vi "hse-application_SetApplicationVersion.vi"(8 "error in":errorcluster, 10 "Application Version History":string, 11 "Application Version Number":string) -> (0 "error out":errorcluster)   [LabVIEW 2020, in "hse-application.lvclass"]
doc: "Stores the version number of the application for later usage (display, logging, ...).\n\n\n\n____\nHAMPEL SOFTWARE ENGINEERING v3.8.0 (2023-12-18 14:41)"
uses:
  hse-application.lvclass
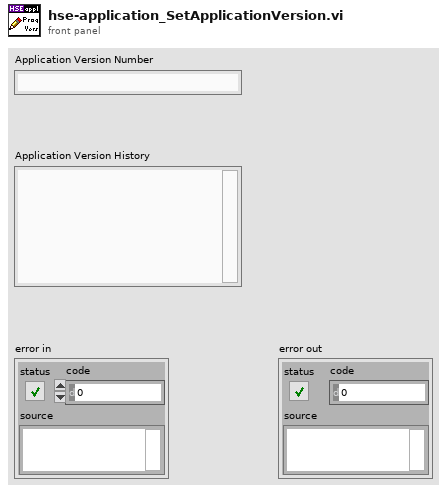
[diagram p1: front panel]
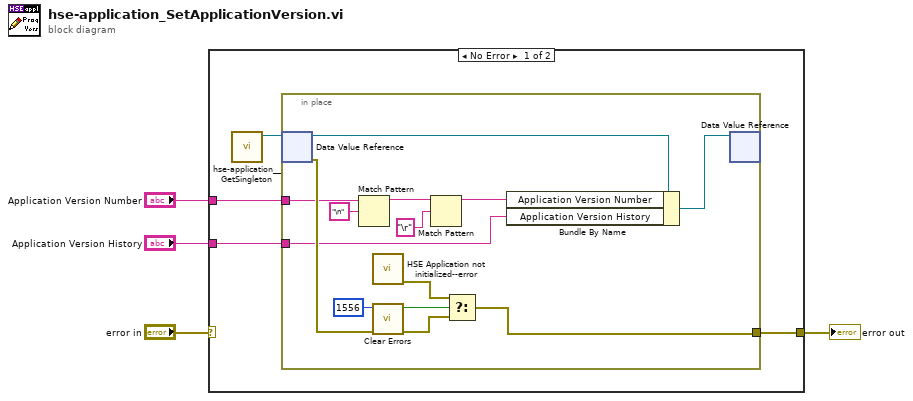
[diagram p0: block diagram]
diagram:
  n1 = case shown="No Error" "error in" {
    selector: "error in" -> [_ w23]
    tunnel: [w8 w23] -> w3
    tunnel: "Application Version Number" -> [w6 _]
    tunnel: "Application Version History" -> [w5 _]
    frame No Error {
      n2 = call "hse-application__GetSingleton.vi"() -> ("ApplicationClass DVR"=w7:refnum<data-value>)  [unwired: 10 in, 1 out]
      n3 = in-place "In Place Element Structure" {
        in-place-border: [w20] -> w8
        in-place-border: w6 -> [w16]
        in-place-border: w5 -> [w15]
        n4 = in-place-dvr #1(w7) -> (w18:refnum<class "hse-application.lvclass">, w19:errorcluster)
        n5 = Match Pattern(string=w16, regular expression="\n") -> (before substring=w12:string)  [unwired: 1 in, 3 out]
        n6 = call "HSE Application not initialized--error.vi"() -> ("error out"=w22:errorcluster)  [unwired: 11 in]
        n7 = call <vilib>:"Clear Errors.vi"("error in (no error)"=w19, "specific error code to clear (0: all)"=1556) -> ("error out"=w21:errorcluster, "specific error cleared?"=w9:bool)  [unwired: 4 in]
        n8 = Match Pattern(string=w12, regular expression="\r") -> (before substring=w11:string)  [unwired: 1 in, 3 out]
        n9 = Select(t=w22, s=w9, f=w21) -> (s? t:f=w20:errorcluster)
        n10 = Bundle By Name(cluster=w18, "Application Version Number"=w11, "Application Version History"=w15) -> (w14:refnum<class "hse-application.lvclass">)
        n11 = in-place-dvr #1(w14) -> ()  [unwired: 2 out]
      }
    }
    frame Error {
    }
  }
  "error out" <- w3
